vi "Profile Auton - Shooting Mode.vi"(8 "error in (no error)":errorcluster, 10 "Time (s)":dbl, 11 "Shooting Mode":T1(ring)) -> (0 "error out":errorcluster)   [LabVIEW 2017]
uses:
  Robot Global Data.vi
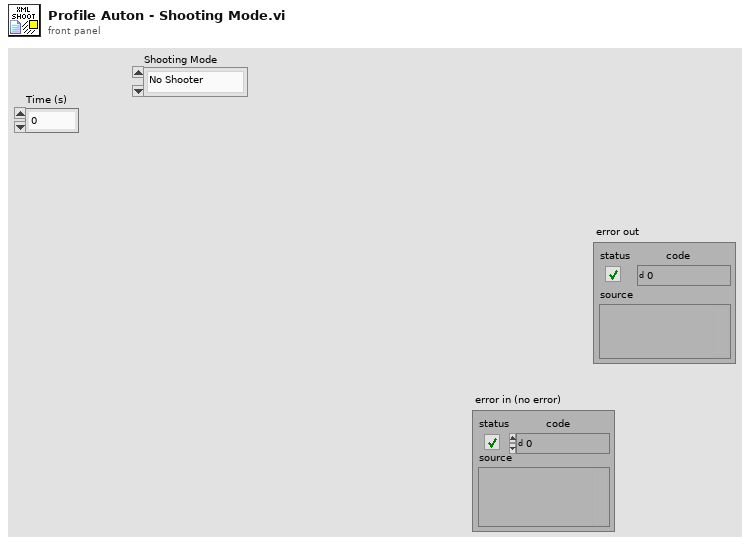
[diagram p1: front panel]
types:
  T1 = enum16{"No Shooter", "Switch Shooter", "Low Scale Shooter", "Mid Scale Shooter", "High Scale Shooter"}
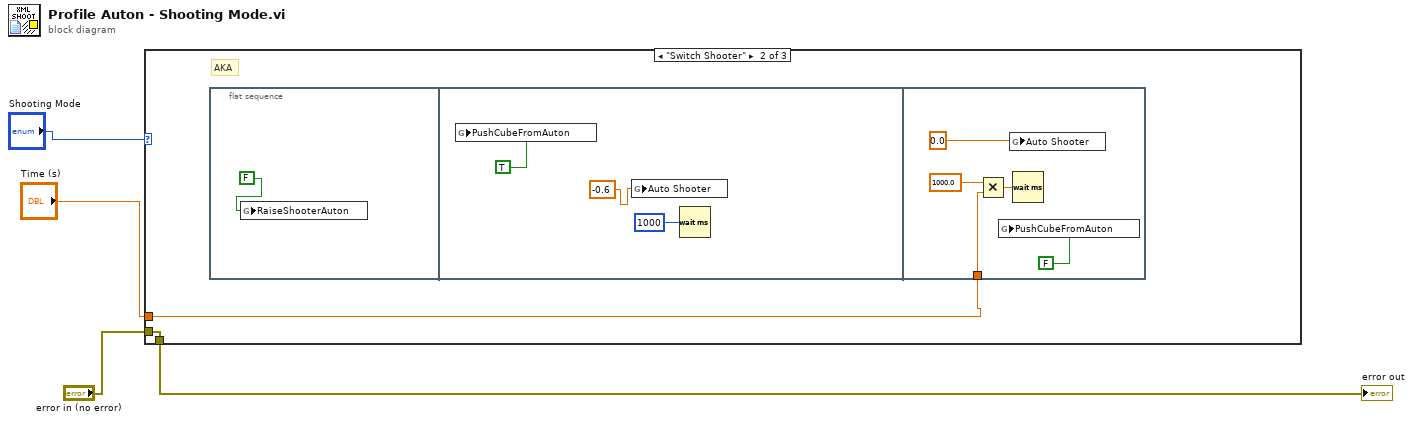
[diagram p0: block diagram]
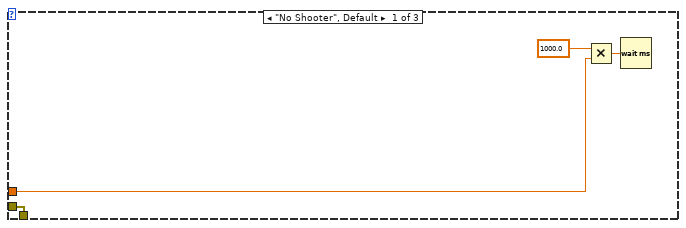
[diagram p2: hidden frame]
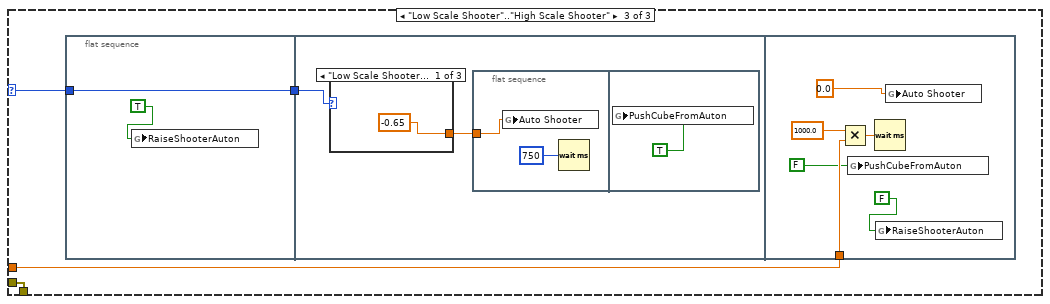
[diagram p3: hidden frame]
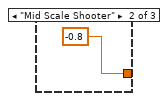
[diagram p4: hidden frame]
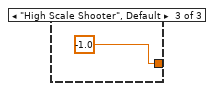
[diagram p5: hidden frame]
diagram:
  n1 = case shown="\"Switch Shooter\"" "Shooting Mode" {
    selector: "Shooting Mode" -> [_ _ w20]
    tunnel: "Time (s)" -> [w6 w10 w23]
    tunnel: "error in (no error)" -> [w5 w9 w22]
    tunnel: [w5 w9 w22] -> w2
    frame "No Shooter", Default {
      n2 = Multiply(x=1000.0, y=w6) -> (x*y=w8:dbl)
      n3 = Wait (ms)(milliseconds to wait=w8) -> ()  [unwired: 1 out]
    }
    frame "Switch Shooter" {
      # "AKA"
      n4 = flat-sequence {
        tunnel: w10 -> [w18]
        frame #0 {
          n5 = global write "Robot Global Data.vi" "RaiseShooterAuton"(FALSE) -> ()
        }
        frame #1 {
          n6 = global write "Robot Global Data.vi" "PushCubeFromAuton"(TRUE) -> ()
          n7 = global write "Robot Global Data.vi" "Auto Shooter"(-0.6) -> ()
          n8 = Wait (ms)(milliseconds to wait=u32 1000) -> ()  [unwired: 1 out]
        }
        frame #2 {
          n9 = Multiply(x=1000.0, y=w18) -> (x*y=w19:dbl)
          n10 = global write "Robot Global Data.vi" "PushCubeFromAuton"(FALSE) -> ()
          n11 = global write "Robot Global Data.vi" "Auto Shooter"(0.0) -> ()
          n12 = Wait (ms)(milliseconds to wait=w19) -> ()  [unwired: 1 out]
        }
      }
    }
    frame "Low Scale Shooter".."High Scale Shooter" {
      n13 = flat-sequence {
        tunnel: [w24] -> w21
        tunnel: w20 -> [w24]
        tunnel: w21 -> [w27]
        tunnel: w23 -> [w38]
        frame #0 {
          n14 = global write "Robot Global Data.vi" "RaiseShooterAuton"(TRUE) -> ()
        }
        frame #1 {
          n15 = case shown="\"Low Scale Shooter\"" w27 {
            tunnel: [-0.65 -0.8 -1.0] -> w26
            frame "Low Scale Shooter" {
            }
            frame "Mid Scale Shooter" {
            }
            frame "High Scale Shooter", Default {
            }
          }
          n16 = flat-sequence {
            tunnel: w26 -> [w31]
            frame #0 {
              n17 = global write "Robot Global Data.vi" "Auto Shooter"(w31) -> ()
              n18 = Wait (ms)(milliseconds to wait=u32 750) -> ()  [unwired: 1 out]
            }
            frame #1 {
              n19 = global write "Robot Global Data.vi" "PushCubeFromAuton"(TRUE) -> ()
            }
          }
        }
        frame #2 {
          n20 = Multiply(x=1000.0, y=w38) -> (x*y=w39:dbl)
          n21 = global write "Robot Global Data.vi" "PushCubeFromAuton"(FALSE) -> ()
          n22 = Wait (ms)(milliseconds to wait=w39) -> ()  [unwired: 1 out]
          n23 = global write "Robot Global Data.vi" "RaiseShooterAuton"(FALSE) -> ()
          n24 = global write "Robot Global Data.vi" "Auto Shooter"(0.0) -> ()
        }
      }
    }
  }
  "error out" <- w2
